vi "TCP&IP_Server_Test.vi"() -> ()   [LabVIEW 2017]
panel:
  in  "Exit":bool
  in  "WriteData":bool
  in  "写入数据":string
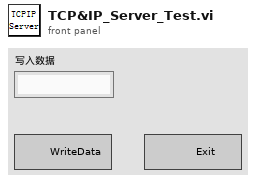
[diagram p1: front panel]
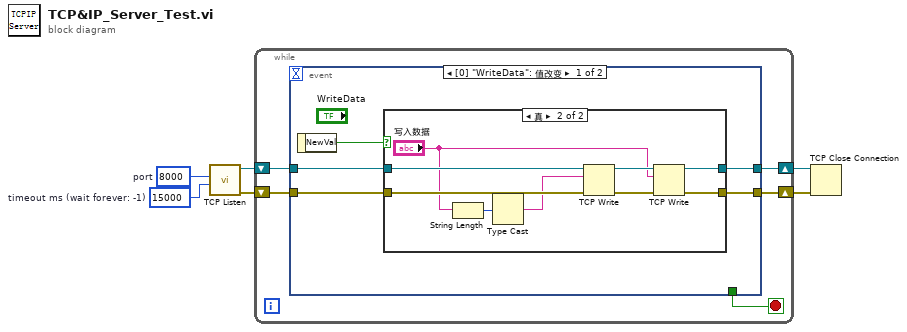
[diagram p0: block diagram]
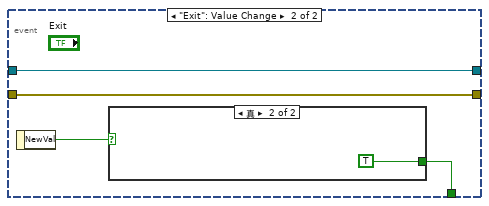
[diagram p3: hidden frame]
diagram:
  w5 = 15000  # timeout ms (wait forever: -1)
  w6 = u16 8000  # port
  n1 = call <vilib>:"TCP Listen.vi"("timeout ms (wait forever: -1)"=w5, "port"=w6) -> ("error out"=w3:errorcluster, "connection ID"=w4:refnum<k5>)  [unwired: 5 in, 3 out]
  n2 = while {
    shift-right: [w10] -> w1
    shift-left: w4 -> [w9]
    shift-right: [w11] -> w2
    shift-left: w3 -> [w8]
    stop <- w7 stop-if-true
    n3 = event shown="[0] \"WriteData\": 值改变" {
      selector: _ -> [_ _]
      dyn-events: _ -> [_ _]
      timeout: _ -> [_ _]
      tunnel: [w16 w29] -> w11
      tunnel: [w15 w30] -> w10
      tunnel: w9 -> [w14 w30]
      tunnel: w8 -> [w13 w29]
      tunnel: [_ w28] -> w7
      event "WriteData": Value Change {
        n4 = event-data() -> ("NewVal"=w12:bool)  [unwired: 1 in]
        n5 = case shown="真" w12 {
          tunnel: [w17 w27] -> w16
          tunnel: [w18 w26] -> w15
          tunnel: w14 -> [w18 w25]
          tunnel: w13 -> [w17 w23]
          frame False {
          }
          frame True {
            n6 = String Length(string="写入数据") -> (length=w21:i32)
            n7 = Type Cast(x=w21) -> (*(type *) &x=w20:string)  [unwired: 1 in]
            n8 = TCP Write ("写入TCP数据")(connection ID=w25, data in=w20, error in (no error)=w23) -> (connection ID out=w24:refnum<k5>, error out=w22:errorcluster)  [unwired: 1 in, 1 out]
            n9 = TCP Write ("写入TCP数据")(connection ID=w24, data in="写入数据", error in (no error)=w22) -> (connection ID out=w26:refnum<k5>, error out=w27:errorcluster)  [unwired: 1 in, 1 out]
          }
        }
      }
      event "Exit": Value Change {
        n10 = event-data() -> ("NewVal"=w31:bool)  [unwired: 1 in]
        n11 = case shown="真" w31 {
          tunnel: [_ TRUE] -> w28
          frame False {
          }
          frame True {
          }
        }
      }
    }
  }
  n12 = TCP Close Connection(connection ID=w1, error in (no error)=w2) -> ()  [unwired: 1 in, 2 out]
